vi "Init.vi"(8 "error in (no error)":errorcluster) -> (0 "error out":errorcluster, 1 "DAQ Queue":refnum<queue>)   [LabVIEW 2017]
doc: "Initialize VI"
uses:
  DAQ States.ctl
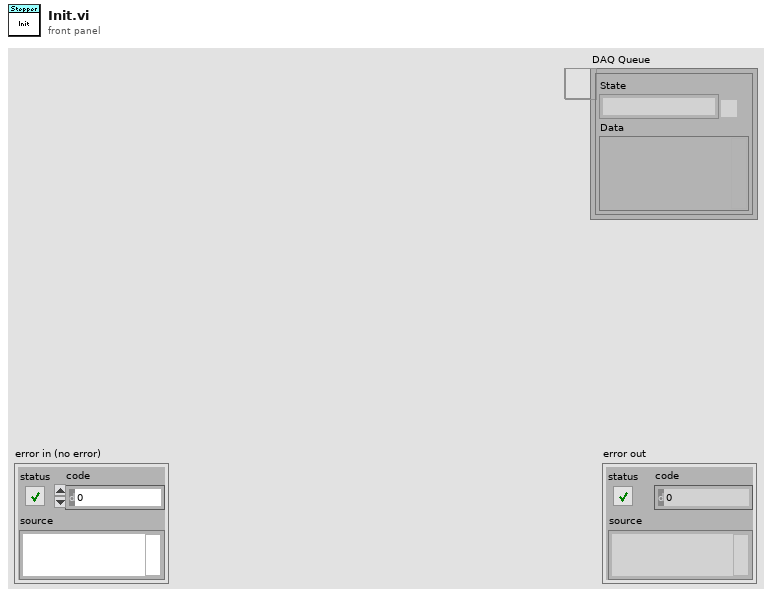
[diagram p1: front panel]
types:
  T1 = typedef "DAQ States.ctl" = enum16{"Init", "Exit", "Update Settings", "Pause", "Update Square", "Update Duration"}
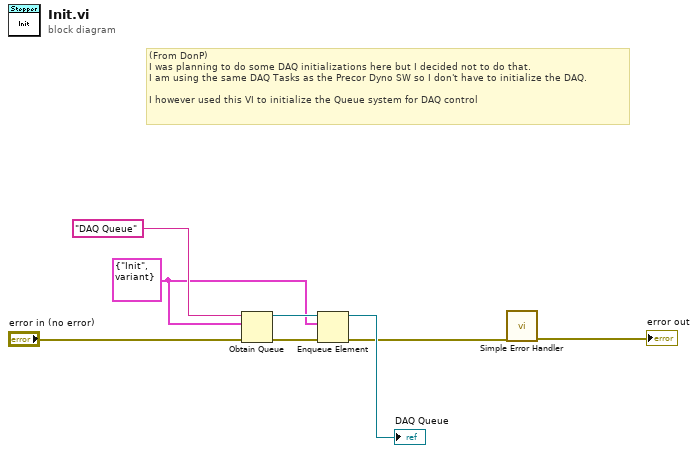
[diagram p0: block diagram]
diagram:
  w4 = cluster{"State":T1, "Data":variant} {"State"=enum."Init", "Data"=variant} ("DAQ Queue")
  # "(From DonP)\nI was planning to do some DAQ initializations here but I decided not to do that.\nI am using the same DAQ Tasks as the Precor Dyno SW so I don't have to initialize the DAQ.\n\nI however used this VI to initialize the Queue system for DAQ control"
  n1 = Obtain Queue(name (unnamed)="DAQ Queue", element data type=w4, error in (no error)="error in (no error)") -> (queue out=w6:refnum<queue>, error out=w5:errorcluster)  [unwired: 2 in, 1 out]
  n2 = Enqueue Element(queue=w6, element=w4, error in (no error)=w5) -> (queue out=→"DAQ Queue":refnum<queue>, error out=w2:errorcluster)  [unwired: 1 in, 1 out]
  n3 = call <vilib>:"Simple Error Handler.vi"("error in (no error)"=w2) -> ("error out"=→"error out":errorcluster)  [unwired: 4 in, 4 out]
